vi "TEST - Slice 1D Array.vi"(8 "error in (no error)":errorcluster) -> (0 "error out":errorcluster, 2 "Pass?":bool=TRUE)   [LabVIEW 2009]
doc: "This VI template can be used for the functional testing of VIs; this implementation includes handling for the testing of polymorphic VIs, and the polymorphic elements should be removed if not needed.\n\nCoded by Douglas A. Femec, January 24, 2006.\n\nCopyright (c) 2005-2006 MKS Instruments, Inc.\nAll rights reserved."
uses:
  TEST - Slice 1D Array - Inputs.ctl
  Polymorphizer+ Data Type.ctl
  TEST - Slice 1D Array - Outputs.ctl
  source/library/Slice 1D Array/Slice 1D Array (EXT).vi
  source/library/Slice 1D Array/Slice 1D Array (I64).vi
  source/library/Slice 1D Array/Slice 1D Array (U64).vi
  source/library/Slice 1D Array/Slice 1D Array (LVObject).vi
  source/library/Slice 1D Array/Slice 1D Array (DBL).vi
  source/library/Slice 1D Array/Slice 1D Array (SIG).vi
  source/library/Slice 1D Array/Slice 1D Array (I32).vi
  source/library/Slice 1D Array/Slice 1D Array (I16).vi
  source/library/Slice 1D Array/Slice 1D Array (I08).vi
  source/library/Slice 1D Array/Slice 1D Array (U32).vi
  source/library/Slice 1D Array/Slice 1D Array (U16).vi
  source/library/Slice 1D Array/Slice 1D Array (U08).vi
  source/library/Slice 1D Array/Slice 1D Array (CXT).vi
  source/library/Slice 1D Array/Slice 1D Array (CDB).vi
  source/library/Slice 1D Array/Slice 1D Array (CSG).vi
  source/library/Slice 1D Array/Slice 1D Array (BOL).vi
  source/library/Slice 1D Array/Slice 1D Array (String).vi
  source/library/Slice 1D Array/Slice 1D Array (PATH).vi
  source/library/Slice 1D Array/Slice 1D Array (VAR).vi
  source/library/Slice 1D Array/Slice 1D Array (CTL-REF).vi
  source/library/Slice 1D Array/Slice 1D Array (ENUM).vi
  source/library/Slice 1D Array/Slice 1D Array (ERR).vi
  source/library/Slice 1D Array/Slice 1D Array (FILE-REF).vi
  source/library/Slice 1D Array/Slice 1D Array (MENU-REF).vi
  source/library/Slice 1D Array/Slice 1D Array (MENU-RING).vi
  source/library/Slice 1D Array/Slice 1D Array (PICT-RING).vi
  source/library/Slice 1D Array/Slice 1D Array (TXT&PICT-RING).vi
  source/library/Slice 1D Array/Slice 1D Array (TXT-RING).vi
  TestClass/TestClass.lvclass
panel:
  in  "Byte Stream File Refnum":refnum<file>
  in  "Ctl Refnum":refnum<vi>
  in  "Menu Refnum":refnum<k9>
  out "Generated Outputs":T1[][](array[typedef]) {"Array Slice Out" format="%.2f"}
  in  "Expected Outputs":T1[](array[typedef])=[{"Description"="Expect empty array", "Array Slice Out"=[]}, {"Description"="Expect empty array", "Array Slice Out"=[]}, {"Description"="Expect empty array", "Array Slice Out"=[]}, {"Description"="Expect one-element array", "Array Slice Out"=[1.0]}, {"Description"="Expect empty array", "Array Slice Out"=[]}, {"Description"="Expect empty array", "Array Slice Out"=[]}, {"Description"="Expect two-element array", "Array Slice Out"=[1.0, 0.0]}, {"Description"="Expect empty array", "Array Slice Out"=[]}, {"Description"="Expect empty array", "Array Slice Out"=[]}, {"Description"="Expect two-element array", "Array Slice Out"=[0.0, 1.0]}, {"Description"="Expect one-element array", "Array Slice Out"=[0.0]}] {"Array Slice Out" format="%.2f"}
  in  "Inputs":T2[](array[typedef])=[{"Description"="Empty array, requesting no net elements", "Data Types to Test"=[enum."EXT", enum."DBL", enum."SGL", enum."I32", enum."I16", enum."I8", enum."U32", enum."U16", enum."U8", enum."CXT", enum."CDB", enum."CSG", enum."Boolean", enum."String", enum."Path", enum."Variant", enum."CTL-REF", enum."ENUM", enum."ERR", enum."FILE-REF", enum."MENU-REF", enum."MENU-RING", enum."PICT-RING", enum."TXT&PICT-RING", enum."TXT-RING", enum."I64", enum."U64", enum."LabVIEW Object"], "Array In"=[], "slice"="0:0"}, {"Description"="Empty array, requesting one net element", "Data Types to Test"=[enum."EXT", enum."DBL", enum."SGL", enum."I32", enum."I16", enum."I8", enum."U32", enum."U16", enum."U8", enum."CXT", enum."CDB", enum."CSG", enum."Boolean", enum."String", enum."Path", enum."Variant", enum."CTL-REF", enum."ENUM", enum."ERR", enum."FILE-REF", enum."MENU-REF", enum."MENU-RING", enum."PICT-RING", enum."TXT&PICT-RING", enum."TXT-RING", enum."I64", enum."U64", enum."LabVIEW Object"], "Array In"=[], "slice"="4:5"}, {"Description"="One-element array, requesting no net elements", "Data Types to Test"=[enum."EXT", enum."DBL", enum."SGL", enum."I32", enum."I16", enum."I8", enum."U32", enum."U16", enum."U8", enum."CXT", enum."CDB", enum."CSG", enum."Boolean", enum."String", enum."Path", enum."Variant", enum."CTL-REF", enum."ENUM", enum."ERR", enum."FILE-REF", enum."MENU-REF", enum."MENU-RING", enum."PICT-RING", enum."TXT&PICT-RING", enum."TXT-RING", enum."I64", enum."U64", enum."LabVIEW Object"], "Array In"=[1.0], "slice"="0:0"}, {"Description"="One-element array, requesting top element", "Data Types to Test"=[enum."EXT", enum."DBL", enum."SGL", enum."I32", enum."I16", enum."I8", enum."U32", enum."U16", enum."U8", enum."CXT", enum."CDB", enum."CSG", enum."Boolean", enum."String", enum."Path", enum."Variant", enum."CTL-REF", enum."ENUM", enum."ERR", enum."FILE-REF", enum."MENU-REF", enum."MENU-RING", enum."PICT-RING", enum."TXT&PICT-RING", enum."TXT-RING", enum."I64", enum."U64", enum."LabVIEW Object"], "Array In"=[1.0], "slice"="0:1"}, {"Description"="One-element array, requesting one net element", "Data Types to Test"=[enum."EXT", enum."DBL", enum."SGL", enum."I32", enum."I16", enum."I8", enum."U32", enum."U16", enum."U8", enum."CXT", enum."CDB", enum."CSG", enum."Boolean", enum."String", enum."Path", enum."Variant", enum."CTL-REF", enum."ENUM", enum."ERR", enum."FILE-REF", enum."MENU-REF", enum."MENU-RING", enum."PICT-RING", enum."TXT&PICT-RING", enum."TXT-RING", enum."I64", enum."U64", enum."LabVIEW Object"], "Array In"=[1.0], "slice"="4:5"}, {"Description"="Three-element array, requesting no net elements", "Data Types to Test"=[enum."EXT", enum."DBL", enum."SGL", enum."I32", enum."I16", enum."I8", enum."U32", enum."U16", enum."U8", enum."CXT", enum."CDB", enum."CSG", enum."Boolean", enum."String", enum."Path", enum."Variant", enum."CTL-REF", enum."ENUM", enum."ERR", enum."FILE-REF", enum."MENU-REF", enum."MENU-RING", enum."PICT-RING", enum."TXT&PICT-RING", enum."TXT-RING", enum."I64", enum."U64", enum."LabVIEW Object"], "Array In"=[1.0, 1.0, 0.0], "slice"="0:0"}, {"Description"="Three-element array, requesting middle two net elements", "Data Types to Test"=[enum."EXT", enum."DBL", enum."SGL", enum."I32", enum."I16", enum."I8", enum."U32", enum."U16", enum."U8", enum."CXT", enum."CDB", enum."CSG", enum."Boolean", enum."String", enum."Path", enum."Variant", enum."CTL-REF", enum."ENUM", enum."ERR", enum."FILE-REF", enum."MENU-REF", enum."MENU-RING", enum."PICT-RING", enum."TXT&PICT-RING", enum."TXT-RING", enum."I64", enum."U64", enum."LabVIEW Object"], "Array In"=[1.0, 1.0, 0.0], "slice"="1:3"}, {"Description"="Three-element array, requesting one net element", "Data Types to Test"=[enum."EXT", enum."DBL", enum."SGL", enum."I32", enum."I16", enum."I8", enum."U32", enum."U16", enum."U8", enum."CXT", enum."CDB", enum."CSG", enum."Boolean", enum."String", enum."Path", enum."Variant", enum."CTL-REF", enum."ENUM", enum."ERR", enum."FILE-REF", enum."MENU-REF", enum."MENU-RING", enum."PICT-RING", enum."TXT&PICT-RING", enum."TXT-RING", enum."I64", enum."U64", enum."LabVIEW Object"], "Array In"=[1.0, 1.0, 0.0], "slice"="4:5"}, {"Description"="Five-element array, requesting no net elements", "Data Types to Test"=[enum."EXT", enum."DBL", enum."SGL", enum."I32", enum."I16", enum."I8", enum."U32", enum."U16", enum."U8", enum."CXT", enum."CDB", enum."CSG", enum."Boolean", enum."String", enum."Path", enum."Variant", enum."CTL-REF", enum."ENUM", enum."ERR", enum."FILE-REF", enum."MENU-REF", enum."MENU-RING", enum."PICT-RING", enum."TXT&PICT-RING", enum."TXT-RING", enum."I64", enum."U64", enum."LabVIEW Object"], "Array In"=[0.0, 0.0, 1.0, 1.0, 0.0], "slice"="0:0"}, {"Description"="Five-element array, requesting middle two net elements", "Data Types to Test"=[enum."EXT", enum."DBL", enum."SGL", enum."I32", enum."I16", enum."I8", enum."U32", enum."U16", enum."U8", enum."CXT", enum."CDB", enum."CSG", enum."Boolean", enum."String", enum."Path", enum."Variant", enum."CTL-REF", enum."ENUM", enum."ERR", enum."FILE-REF", enum."MENU-REF", enum."MENU-RING", enum."PICT-RING", enum."TXT&PICT-RING", enum."TXT-RING", enum."I64", enum."U64", enum."LabVIEW Object"], "Array In"=[0.0, 0.0, 1.0, 1.0, 0.0], "slice"="1:3"}, {"Description"="Five-element array, requesting one net element", "Data Types to Test"=[enum."EXT", enum."DBL", enum."SGL", enum."I32", enum."I16", enum."I8", enum."U32", enum."U16", enum."U8", enum."CXT", enum."CDB", enum."CSG", enum."Boolean", enum."String", enum."Path", enum."Variant", enum."CTL-REF", enum."ENUM", enum."ERR", enum."FILE-REF", enum."MENU-REF", enum."MENU-RING", enum."PICT-RING", enum."TXT&PICT-RING", enum."TXT-RING", enum."I64", enum."U64", enum."LabVIEW Object"], "Array In"=[0.0, 0.0, 1.0, 1.0, 0.0], "slice"="4:5"}] {"Array In" format="%.2f"}
  # "Copyright (c) 2005-2006 MKS Instruments, Inc.\nAll rights reserved."
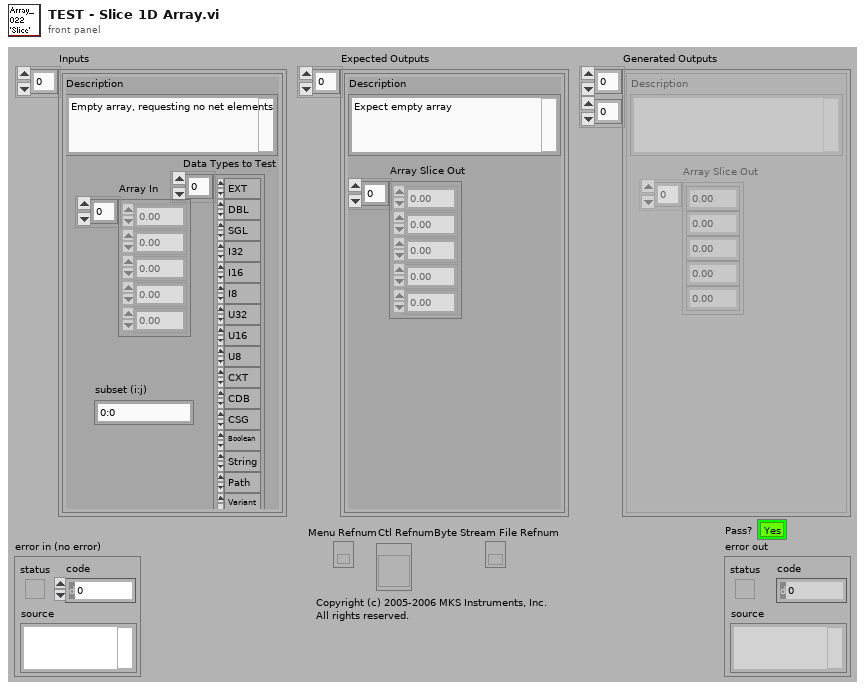
[diagram p1: front panel]
types:
  T1 = typedef "TEST - Slice 1D Array - Outputs.ctl" = cluster{"Description":string, "Array Slice Out":sgl[]}
  T2 = typedef "TEST - Slice 1D Array - Inputs.ctl" = cluster{"Description":string, "Data Types to Test":T3[], "Array In":sgl[], "slice":string}
  T3 = typedef "Polymorphizer+ Data Type.ctl" = enum16{"EXT", "DBL", "SGL", "I32", "I16", "I8", "U32", "U16", "U8", "CXT", "CDB", "CSG", "Boolean", "String", "Path", "Variant", "CTL-REF", "GEN-REF", "GObj-REF", "VI-REF", "ENUM", "ERR", "FILE-REF", "MENU-REF", "MENU-RING", "PICT-RING", "TXT&PICT-RING", "TXT-RING", "I64", "U64", "LabVIEW Object"}
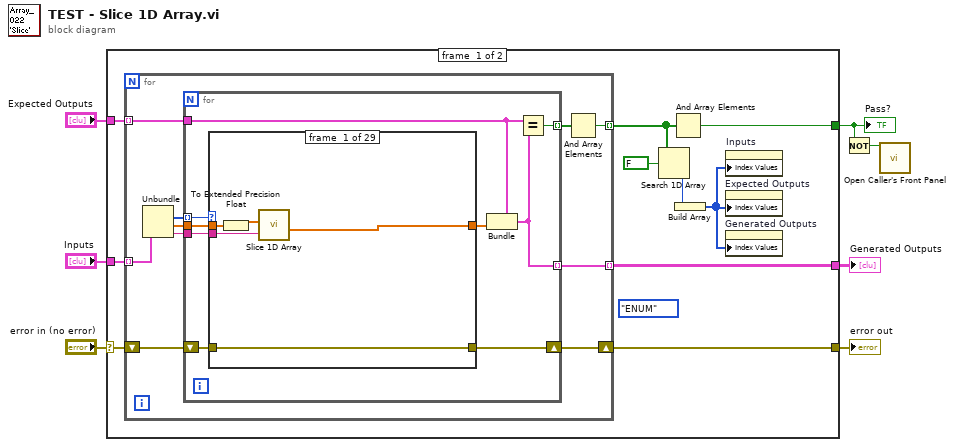
[diagram p0: block diagram]
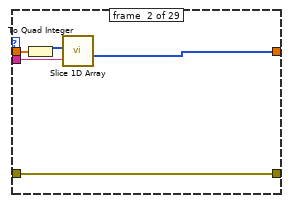
[diagram p2: hidden frame]
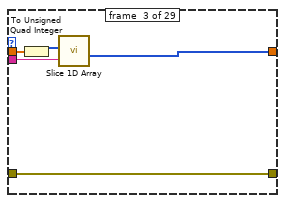
[diagram p3: hidden frame]
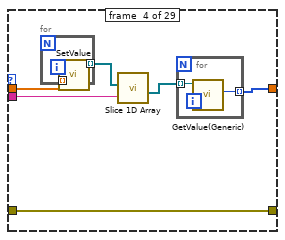
[diagram p4: hidden frame]
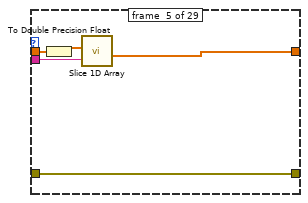
[diagram p5: hidden frame]
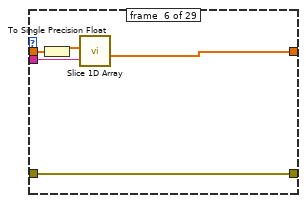
[diagram p6: hidden frame]
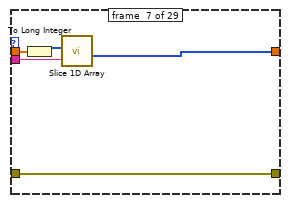
[diagram p7: hidden frame]
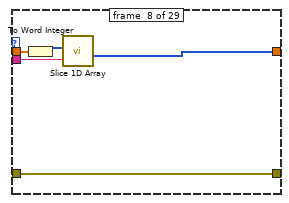
[diagram p8: hidden frame]
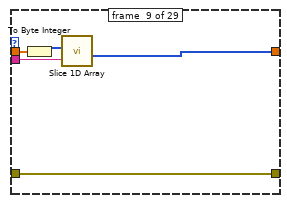
[diagram p9: hidden frame]
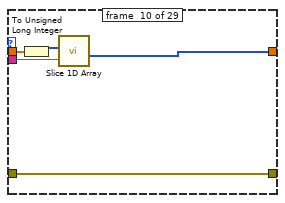
[diagram p10: hidden frame]
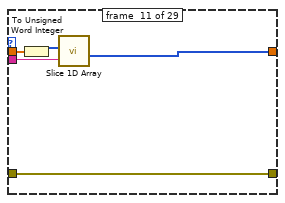
[diagram p11: hidden frame]
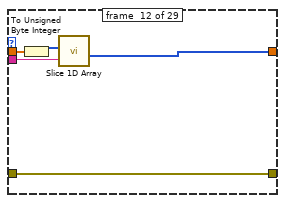
[diagram p12: hidden frame]
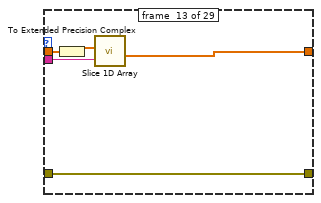
[diagram p13: hidden frame]
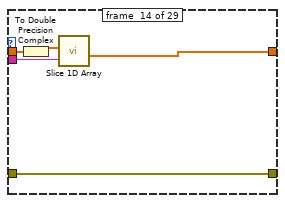
[diagram p14: hidden frame]
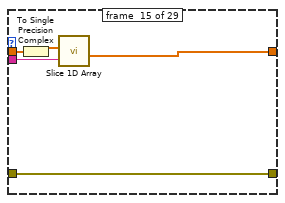
[diagram p15: hidden frame]
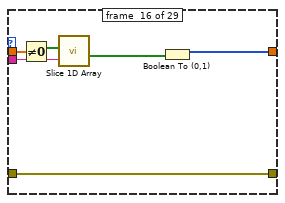
[diagram p16: hidden frame]
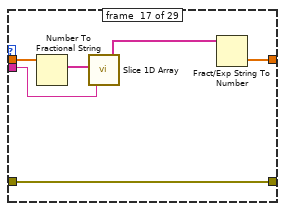
[diagram p17: hidden frame]
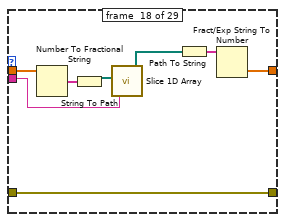
[diagram p18: hidden frame]
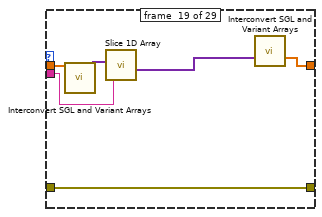
[diagram p19: hidden frame]
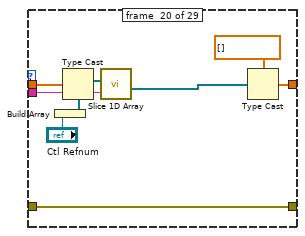
[diagram p20: hidden frame]
diagram:
  n1 = case shown="No Error" "error in (no error)" {
    selector: "error in (no error)" -> [w16 w217]
    tunnel: [w17 w217] -> w6
    tunnel: "Expected Outputs" -> [w14 _]
    tunnel: "Inputs" -> [w15 _]
    tunnel: [w13 _] -> w3
    tunnel: [w12 _] -> w2
    frame #0 {
      (unwired) Polymorphizer+_Data_Type."ENUM" ("Data Type")
      n2 = for {
        shift-right: [w22] -> w17
        shift-left: w16 -> [w23]
        tunnel: w15 -> [w24] mode=indexing
        tunnel: w14 -> [w27] mode=indexing
        tunnel: [w26] -> w13 mode=indexing
        tunnel: [w21] -> w11 mode=indexing
        n3 = Unbundle(w24) -> ("Data Types to Test"=w20:T3[], "Array In"=w19:sgl[], "slice"=w18:string)  [unwired: 1 out]
        n4 = for {
          tunnel: w27 -> [w36]
          tunnel: [w34] -> w26 mode=indexing
          tunnel: [w35] -> w25 mode=indexing
          shift-right: [w30] -> w22
          shift-left: w23 -> [w31]
          tunnel: w20 -> [w32] mode=indexing
          tunnel: w19 -> [w33]
          tunnel: w18 -> [w29]
          n5 = case shown="\"LabVIEW Object\"" w32 {
            tunnel: w33 -> [w39 w44 w49 w55 w64 w69 w74 w79 w84 w89 w94 w99 w104 w109 w114 w120 w126 w132 w139 w149 w154 w169 w183 w192 w197 w202 w207 w212 w216]
            tunnel: [w40 w45 w50 w52 w65 w70 w75 w80 w85 w90 w95 w100 w105 w110 w115 w117 w128 w135 w141 w144 w156 w166 w179 w188 w198 w203 w208 w213 w216] -> w28
            tunnel: w31 -> [w41 w46 w51 w57 w66 w71 w76 w81 w86 w91 w96 w101 w106 w111 w116 w122 w127 w133 w142 w151 w157 w170 w185 w194 w199 w204 w209 w214 w215]
            tunnel: [w41 w46 w51 w57 w66 w71 w76 w81 w86 w91 w96 w101 w106 w111 w116 w122 w127 w133 w142 w151 w157 w170 w185 w194 w199 w204 w209 w214 w215] -> w30
            tunnel: w29 -> [w37 w42 w47 w56 w62 w67 w72 w77 w82 w87 w92 w97 w102 w107 w112 w118 w124 w129 w137 w147 w152 w171 w181 w190 w195 w200 w205 w210 _]
            frame #0 {
              n6 = To Extended Precision Float(1:w39) -> (0:w38:ext[])
              n7 = call-poly "Slice 1D Array.vi"("slice"=w37, "array"=w38) -> ("subarray (array[i:j])"=w40:ext[])  [unwired: 5 in]
            }
            frame #1 {
              n8 = To Quad Integer(1:w44) -> (0:w43:i64[])
              n9 = call-poly "Slice 1D Array.vi"("slice"=w42, "array"=w43) -> ("subarray (array[i:j])"=w45:i64[])  [unwired: 5 in]
            }
            frame #2 {
              n10 = To Unsigned Quad Integer(1:w49) -> (0:w48:u64[])
              n11 = call-poly "Slice 1D Array.vi"("slice"=w47, "array"=w48) -> ("subarray (array[i:j])"=w50:u64[])  [unwired: 5 in]
            }
            frame #3 {
              n12 = for {
                tunnel: w55 -> [w59] mode=indexing
                tunnel: [w58] -> w54 mode=indexing
                n13 = call "SetValue.vi"("Value"=w59) -> ("TestClass out"=w58:refnum<class "TestClass.lvclass">)  [unwired: 9 in, 1 out]
              }
              n14 = call-poly "Slice 1D Array.vi"("slice"=w56, "array"=w54) -> ("subarray (array[i:j])"=w53:refnum<class>[])  [unwired: 5 in]
              n15 = for {
                tunnel: w53 -> [w61] mode=indexing
                tunnel: [w60] -> w52 mode=indexing
                n16 = call "GetValue(Generic).vi"("TestClass in"=w61) -> ("Value"=w60:i32)  [unwired: 8 in, 2 out]
              }
            }
            frame #4 {
              n17 = To Double Precision Float(number=w64) -> (double precision float=w63:dbl[])
              n18 = call-poly "Slice 1D Array.vi"("slice"=w62, "array"=w63) -> ("subarray (array[i:j])"=w65:dbl[])  [unwired: 5 in]
            }
            frame #5 {
              n19 = To Single Precision Float(number=w69) -> (single precision float=w68:sgl[])
              n20 = call-poly "Slice 1D Array.vi"("slice"=w67, "array"=w68) -> ("subarray (array[i:j])"=w70:sgl[])  [unwired: 5 in]
            }
            frame #6 {
              n21 = To Long Integer(number=w74) -> (32bit integer=w73:i32[])
              n22 = call-poly "Slice 1D Array.vi"("slice"=w72, "array"=w73) -> ("subarray (array[i:j])"=w75:i32[])  [unwired: 5 in]
            }
            frame #7 {
              n23 = To Word Integer(number=w79) -> (16bit integer=w78:i16[])
              n24 = call-poly "Slice 1D Array.vi"("slice"=w77, "array"=w78) -> ("subarray (array[i:j])"=w80:i16[])  [unwired: 5 in]
            }
            frame #8 {
              n25 = To Byte Integer(number=w84) -> (8bit integer=w83:i8[])
              n26 = call-poly "Slice 1D Array.vi"("slice"=w82, "array"=w83) -> ("subarray (array[i:j])"=w85:i8[])  [unwired: 5 in]
            }
            frame #9 {
              n27 = To Unsigned Long Integer(number=w89) -> (unsigned 32bit integer=w88:u32[])
              n28 = call-poly "Slice 1D Array.vi"("slice"=w87, "array"=w88) -> ("subarray (array[i:j])"=w90:u32[])  [unwired: 5 in]
            }
            frame #10 {
              n29 = To Unsigned Word Integer(number=w94) -> (unsigned 16bit integer=w93:u16[])
              n30 = call-poly "Slice 1D Array.vi"("slice"=w92, "array"=w93) -> ("subarray (array[i:j])"=w95:u16[])  [unwired: 5 in]
            }
            frame #11 {
              n31 = To Unsigned Byte Integer(number=w99) -> (unsigned 8bit integer=w98:u8[])
              n32 = call-poly "Slice 1D Array.vi"("slice"=w97, "array"=w98) -> ("subarray (array[i:j])"=w100:u8[])  [unwired: 5 in]
            }
            frame #12 {
              n33 = To Extended Precision Complex(1:w104) -> (0:w103:cxt[])
              n34 = call-poly "Slice 1D Array.vi"("slice"=w102, "array"=w103) -> ("subarray (array[i:j])"=w105:cxt[])  [unwired: 5 in]
            }
            frame #13 {
              n35 = To Double Precision Complex(1:w109) -> (0:w108:cdb[])
              n36 = call-poly "Slice 1D Array.vi"("slice"=w107, "array"=w108) -> ("subarray (array[i:j])"=w110:cdb[])  [unwired: 5 in]
            }
            frame #14 {
              n37 = To Single Precision Complex(1:w114) -> (0:w113:csg[])
              n38 = call-poly "Slice 1D Array.vi"("slice"=w112, "array"=w113) -> ("subarray (array[i:j])"=w115:csg[])  [unwired: 5 in]
            }
            frame #15 {
              n39 = Not Equal To 0?(x=w120) -> (x != 0?=w119:bool[])
              n40 = call-poly "Slice 1D Array.vi"("slice"=w118, "array"=w119) -> ("subarray (array[i:j])"=w121:bool[])  [unwired: 5 in]
              n41 = Boolean To (0,1)(Boolean=w121) -> (0, 1=w117:i16[])
            }
            frame #16 {
              n42 = Number To Fractional String(number=w126) -> (F-format string=w125:string[])  [unwired: 3 in]
              n43 = call-poly "Slice 1D Array.vi"("slice"=w124, "array"=w125) -> ("subarray (array[i:j])"=w123:string[])  [unwired: 5 in]
              n44 = Fract/Exp String To Number(string=w123) -> (number=w128:dbl[])  [unwired: 3 in, 1 out]
            }
            frame #17 {
              n45 = Number To Fractional String(number=w132) -> (F-format string=w136:string[])  [unwired: 3 in]
              n46 = String To Path(string=w136) -> (path=w131:path[])
              n47 = call-poly "Slice 1D Array.vi"("slice"=w129, "array"=w131) -> ("subarray (array[i:j])"=w130:path[])  [unwired: 5 in]
              n48 = Path To String(path=w130) -> (string=w134:string[])
              n49 = Fract/Exp String To Number(string=w134) -> (number=w135:dbl[])  [unwired: 3 in, 1 out]
            }
            frame #18 {
              n50 = call "Interconvert SGL and Variant Arrays.vi"("SGL 1D Array In"=w139) -> ("Variant 1D Array Out"=w138:variant[])  [unwired: 10 in, 4 out]
              n51 = call-poly "Slice 1D Array.vi"("slice"=w137, "array"=w138) -> ("subarray (array[i:j])"=w140:variant[])  [unwired: 5 in]
              n52 = call "Interconvert SGL and Variant Arrays.vi"("Variant 1D Array In"=w140) -> ("SGL 1D Array Out"=w141:sgl[])  [unwired: 10 in, 4 out]
            }
            frame #19 {
              n53 = Build Array("Ctl Refnum") -> (w145:refnum<vi>[])
              n54 = Type Cast(type=w145, x=w149) -> (*(type *) &x=w148:refnum<vi>[])
              n55 = call-poly "Slice 1D Array.vi"("slice"=w147, "array"=w148) -> ("subarray (array[i:j])"=w150:refnum<vi>[])  [unwired: 5 in]
              n56 = Type Cast(type=sgl[] [] ("Array Slice Out"), x=w150) -> (*(type *) &x=w144:sgl[])
            }
            frame #20 {
              n57 = for {
                tunnel: w154 -> [w159] mode=indexing
                tunnel: [w158] -> w153 mode=indexing
                n58 = case shown="1" w159 {
                  tunnel: [enum16{"0", "1"}."0" ("Enum") enum16{"0", "1"}."1" ("Enum")] -> w158
                  frame #0 {
                  }
                  frame #1 {
                  }
                }
              }
              n59 = call-poly "Slice 1D Array.vi"("slice"=w152, "array"=w153) -> ("subarray (array[i:j])"=w155:enum16{"0", "1"}[])  [unwired: 5 in]
              n60 = for {
                tunnel: [w164] -> w156 mode=indexing
                tunnel: w155 -> [w165] mode=indexing
                n61 = Format Into String(w165) -> (resulting string=w163:string)  [unwired: 3 in, 1 out]
                n62 = Decimal String To Number(string=w163, default (0L)=sgl 0.0) -> (number=w164:sgl)  [unwired: 1 in, 1 out]
              }
            }
            frame #21 {
              n63 = for {
                tunnel: w170 -> [w176]
                tunnel: w169 -> [w175] mode=indexing
                tunnel: [w174] -> w168 mode=indexing
                n64 = Bundle(cluster=w176, "code"=w175) -> (w174:errorcluster)  [unwired: 2 in]
              }
              n65 = call-poly "Slice 1D Array.vi"("slice"=w171, "array"=w168) -> ("subarray (array[i:j])"=w167:errorcluster[])  [unwired: 5 in]
              n66 = for {
                tunnel: w167 -> [w173] mode=indexing
                tunnel: [w172] -> w166 mode=indexing
                n67 = Unbundle(w173) -> ("code"=w172:i32)  [unwired: 2 out]
              }
            }
            frame #22 {
              n68 = Build Array("Byte Stream File Refnum") -> (w180:refnum<file>[])
              n69 = Type Cast(type=w180, x=w183) -> (*(type *) &x=w182:refnum<file>[])
              n70 = call-poly "Slice 1D Array.vi"("slice"=w181, "array"=w182) -> ("subarray (array[i:j])"=w184:refnum<file>[])  [unwired: 5 in]
              n71 = Type Cast(type=sgl[] [] ("Array Slice Out"), x=w184) -> (*(type *) &x=w179:sgl[])
            }
            frame #23 {
              n72 = Build Array("Menu Refnum") -> (w189:refnum<k9>[])
              n73 = Type Cast(type=w189, x=w192) -> (*(type *) &x=w191:refnum<k9>[])
              n74 = call-poly "Slice 1D Array.vi"("slice"=w190, "array"=w191) -> ("subarray (array[i:j])"=w193:refnum<k9>[])  [unwired: 5 in]
              n75 = Type Cast(type=sgl[] [] ("Array Slice Out"), x=w193) -> (*(type *) &x=w188:sgl[])
            }
            frame #24 {
              n76 = To Unsigned Word Integer(number=w197) -> (unsigned 16bit integer=w196:u16[])
              n77 = call-poly "Slice 1D Array.vi"("slice"=w195, "array"=w196) -> ("subarray (array[i:j])"=w198:u16[])  [unwired: 5 in]
            }
            frame #25 {
              n78 = To Unsigned Word Integer(number=w202) -> (unsigned 16bit integer=w201:u16[])
              n79 = call-poly "Slice 1D Array.vi"("slice"=w200, "array"=w201) -> ("subarray (array[i:j])"=w203:u16[])  [unwired: 5 in]
            }
            frame #26 {
              n80 = To Unsigned Word Integer(number=w207) -> (unsigned 16bit integer=w206:u16[])
              n81 = call-poly "Slice 1D Array.vi"("slice"=w205, "array"=w206) -> ("subarray (array[i:j])"=w208:u16[])  [unwired: 5 in]
            }
            frame #27 {
              n82 = To Unsigned Word Integer(number=w212) -> (unsigned 16bit integer=w211:u16[])
              n83 = call-poly "Slice 1D Array.vi"("slice"=w210, "array"=w211) -> ("subarray (array[i:j])"=w213:u16[])  [unwired: 5 in]
            }
            frame #28 {
            }
          }
          n84 = Bundle(cluster=w36, "Array Slice Out"=w28) -> (w34:T1)  [unwired: 1 in]
          n85 = Equal?(x=w36, y=w34) -> (x = y?=w35:bool)
        }
        n86 = And Array Elements(Boolean array=w25) -> (logical AND=w21:bool)
      }
      n87 = Search 1D Array(1D array=w11, element=FALSE) -> (index of element=w9:i32)  [unwired: 1 in]
      n88 = And Array Elements(Boolean array=w11) -> (logical AND=w12:bool)
      n89 = Build Array(w9) -> (w8:i32[])
      n90 = property on="Inputs" class="Arr (strict)"("Index Values"=w8) -> ()  [unwired: 2 in, 2 out]
      n91 = property on="Expected Outputs" class="Arr (strict)"("Index Values"=w8) -> ()  [unwired: 2 in, 2 out]
      n92 = property on="Generated Outputs" class="Arr (strict)"("Index Values"=w8) -> ()  [unwired: 2 in, 2 out]
    }
    frame #1 {
    }
  }
  "error out" <- w6
  "Pass?" <- w2
  "Generated Outputs" <- w3
  n93 = Not(x=w2) -> (.not. x?=w1:bool)
  n94 = call "Open Caller's Front Panel.vi"("Open?"=w1) -> ()  [unwired: 14 in, 1 out]
